vi "Shoot_wrapper.vi"(8 "otto aline":bool, 9 "wheel":dbl, 10 "turr(et)":dbl, 11 "hood":dbl) -> ()   [LabVIEW 2019]
uses:
  <vilib>/Rock Robotics/WPI/Framework/Command Status Info.ctl
  <vilib>/Rock Robotics/WPI/Framework/Completion Status.ctl
  <vilib>/Rock Robotics/WPI/Framework/Completion Notifier.ctl
panel:
  out "Command Info Out":T1
  in  "Description":string
  in  "Command Info In":T1
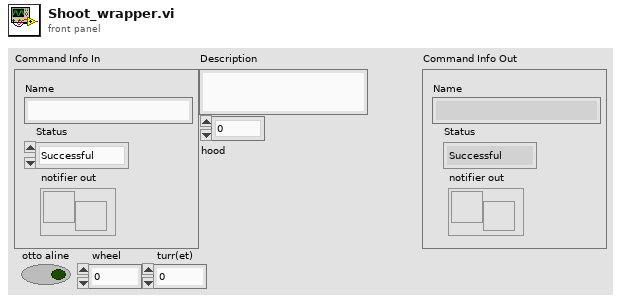
[diagram p1: front panel]
types:
  T1 = typedef "Command Status Info.ctl" = cluster{"Name":string, "Status":T2, "notifier out":T3}
  T2 = typedef "Completion Status.ctl" = enum16{"Successful", "Aborted", "Incomplete"}
  T3 = typedef "Completion Notifier.ctl" = refnum<notifier>
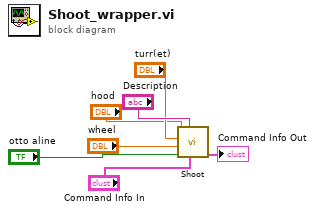
[diagram p0: block diagram]
diagram:
  n1 = call "Shoot.vi"("Command Info In"="Command Info In", "Description"="Description", "otto aline"="otto aline", "wheel"="wheel", "turr(et)"="turr(et)", "hood"="hood") -> ("Command Info Out"=→"Command Info Out":T1)  [unwired: 5 in]
